vi "niRFUtil FTW FFT (complex wfm).vi"(3 "Padding (1)":T1=1.0 min=1.0 format="%.2f", 5 "Waveform In (V)":T2 {"y" format="%.2f"; "dx" format="%^.2e"; "x0" format="%^.2e"}) -> (0 "-ENBW (dB-Hz)":sgl format="%.2f", 1 "Coherent Loss (dB)":sgl format="%.2f", 2 "Waveform Out (V)":T2 {"y" format="%.2f"; "dx" format="%^.2e"; "x0" format="%^.2e"})   [LabVIEW 2015, in "niRFUtil.lvlib"]
doc: "(c) Copyright 2006, National Instruments, Inc. This VI may not be duplicated, sold, or distributed without written consent from National Instruments."
uses:
  niRFUtil.lvlib
  Includes/niRFUtil INC Complex Waveform.ctl
  Includes/niRFUtil INC Complex Array.ctl
  Includes/niRFUtil INC FFT Padding.ctl
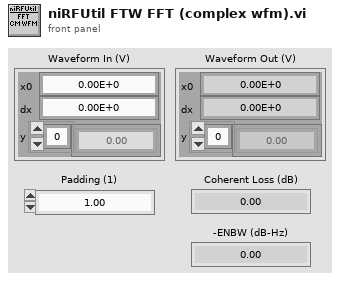
[diagram p1: front panel]
types:
  T1 = typedef "niRFUtil.lvlib/niRFUtil INC FFT Padding.ctl" = dbl
  T2 = typedef "niRFUtil.lvlib/niRFUtil INC Complex Waveform.ctl" = cluster{"x0":dbl, "dx":dbl, "y":T3}
  T3 = typedef "niRFUtil.lvlib/niRFUtil INC Complex Array.ctl" = csg[]
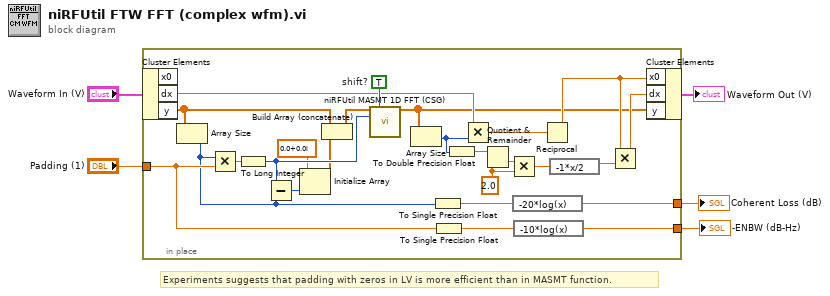
[diagram p0: block diagram]
diagram:
  # "Experiments suggests that padding with zeros in LV is more efficient than in MASMT function."
  n1 = in-place {
    in-place-border: "Padding (1)" -> [w16]
    in-place-border: [w17] -> w2
    in-place-border: [w15] -> w1
    w25 = 2.0 ("y")
    w30 = TRUE  # shift?
    n2 = in-place-cluster #1("Waveform In (V)") -> ("dx"=w24:dbl, "y"=w12:T3)  [unwired: 1 out]
    n3 = Array Size(array=w12) -> (size(s)=w10:i32)
    n4 = Multiply(x=w10, y=w16) -> (x*y=w19:T1)
    n5 = To Long Integer(number=w19) -> (32bit integer=w11:i32)
    n6 = Subtract(x=w11, y=w10) -> (x-y=w9:i32)
    n7 = Initialize Array(csg 0.0+0.0i, w9) -> (w7:csg[])
    n8 = Build Array (concatenate)(w12, w7) -> (w6:T3)
    n9 = call "niRFUtil MASMT 1D FFT (CSG).vi"("X"=w6, "shift?"=w30, "FFT size"=w11) -> ("FFT {X}"=w14:csg[])  [unwired: 11 in, 1 out]
    n10 = Array Size(array=w14) -> (size(s)=w21:i32)
    n11 = To Single Precision Float(number=w10) -> (single precision float=w18:sgl)
    n12 = To Single Precision Float(number=w16) -> (single precision float=w13:sgl)
    n13 = To Double Precision Float(number=w21) -> (double precision float=w20:dbl)
    n14 = Multiply(x=w24, y=w21) -> (x*y=w29:dbl)
    n15 = Quotient & Remainder(x=w20, y=w25) -> (floor(x/y)=w27:dbl)  [unwired: 1 out]
    n16 = Multiply(x=w27, y=w25) -> (x*y=w26:dbl)
    n17 = expression code="-20*log(x)"(w18) -> (w17:sgl)
    n18 = expression code="-10*log(x)"(w13) -> (w15:sgl)
    n19 = Reciprocal(x=w29) -> (1/x=w22:dbl)
    n20 = expression code="-1*x/2"(w26) -> (w28:dbl)
    n21 = Multiply(x=w22, y=w28) -> (x*y=w23:dbl)
    n22 = in-place-cluster #1("x0"=w23, "dx"=w22, "y"=w14) -> (→"Waveform Out (V)":T2)
  }
  "Coherent Loss (dB)" <- w2
  "-ENBW (dB-Hz)" <- w1
